vi "TL_Driver_v2.vi"(0 "Device In":refnum<visa-resource-name>="GPIB0::10::INSTR", 5 "Commands":T1(ring)=enum."SET", 7 "Settings":T3={"Module"=enum."WV Online TEC", "WV Online TEC"=23.204500000000476, "WV Online LD"=0.175, "WV Offline TEC"=29.65925000000015, "WV Offline LD"=0.17, "WV Etalon TEC"=30.6, "HSRL Etalon TEC"=25.954, "HSRL TEC"=14.280749999999731, "HSRL LD"=0.16} {"HSRL LD" min=0.0 max=0.18 step=0.001 format="%.3p"; "HSRL TEC" min=14.0 max=28.0 step=0.1 format="%.3g"; "WV Offline LD" min=0.0 max=0.18 step=0.001 format="%.3p"; "WV Online LD" min=0.0 max=0.18 step=0.001 format="%.3p"; "HSRL Etalon TEC" format="%.2g"; "WV Etalon TEC" format="%.2g"; "WV Offline TEC" min=14.0 max=30.0 step=0.1 format="%.3g"; "WV Online TEC" min=14.0 max=28.0 step=0.1 format="%.3g"}, 11 "error in":errorcluster) -> (4 "Device Out":refnum<visa-resource-name>="GPIB0::10::INSTR", 6 "Response":string, 8 "Readings":T2={"Pro8000"=TRUE, "WV OnLine TEC"=23.2082767, "WV Online TEC"=TRUE, "WV Online LD"=0.175123051, "WV Online LD"=TRUE, "WV Offline TEC"=29.6726017, "WV Offline TEC"=TRUE, "WV Offline LD"=0.170392588, "WV Offline LD"=TRUE, "WV EtalonTEC"=30.5354195, "WV Etalon TEC"=TRUE, "HSRL Etalon TEC"=25.9403496, "HSRL Etalon TEC"=TRUE, "HSRL TEC"=14.2948246, "HSRL TEC "=TRUE, "HSRL LD"=0.160259768, "HSRL LD"=TRUE} {"HSRL LD" format="%.3p"; "HSRL TEC" format="%.3g"; "WV Offline LD" format="%.3p"; "WV Online LD" format="%.3p"; "HSRL Etalon TEC" format="%.3g"; "WV EtalonTEC" format="%.3g"; "WV Offline TEC" format="%.3g"; "WV OnLine TEC" format="%.3g"}, 15 "error out":errorcluster)   [LabVIEW 2012]
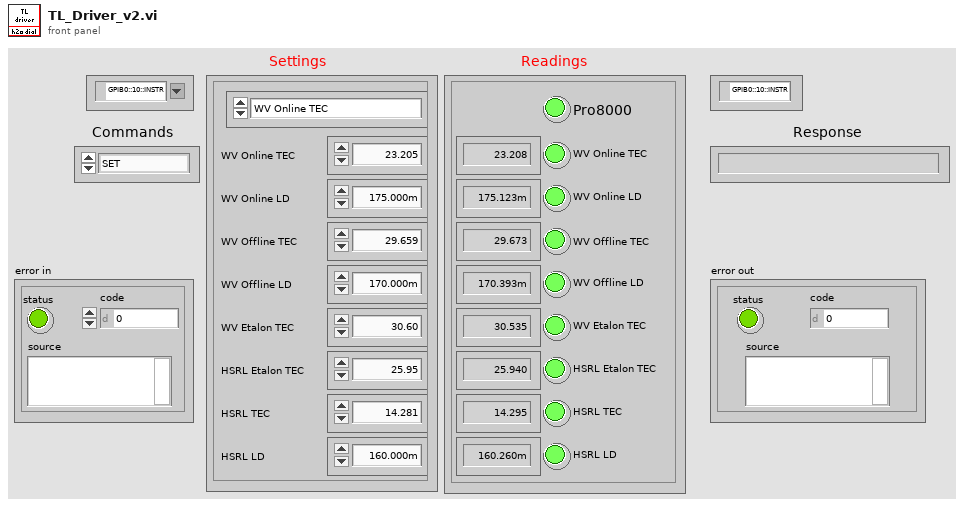
[diagram p1: front panel]
types:
  T1 = enum16{"Open_TL", "Close_TL", "Verify_ID", "TEC_Sensor", "SET", "READ", "ON", "OFF", "Set_Limits", "Read_Limits", "Enable_Status", "Read_Status"}
  T2 = cluster{"Pro8000":bool, "WV OnLine TEC":dbl, "WV Online TEC":bool, "WV Online LD":dbl, "WV Online LD":bool, "WV Offline TEC":dbl, "WV Offline TEC":bool, "WV Offline LD":dbl, "WV Offline LD":bool, "WV EtalonTEC":dbl, "WV Etalon TEC":bool, "HSRL Etalon TEC":dbl, "HSRL Etalon TEC":bool, "HSRL TEC":dbl, "HSRL TEC ":bool, "HSRL LD":dbl, "HSRL LD":bool}
  T3 = cluster{"Module":enum16{"WV Online TEC", "WV Online LD", "WV Offline TEC", "WV Offline LD", "WV Etalon TEC", "HSRL Etalon TEC", "HSRL TEC", "HSRL LD"}, "WV Online TEC":dbl, "WV Online LD":dbl, "WV Offline TEC":dbl, "WV Offline LD":dbl, "WV Etalon TEC":dbl, "HSRL Etalon TEC":dbl, "HSRL TEC":dbl, "HSRL LD":dbl}
  T4 = enum16{"WV Online TEC", "WV Online LD", "WV Offline TEC", "WV Offline LD", "WV Etalon TEC", "HSRL Etalon TEC", "HSRL TEC", "HSRL LD"}
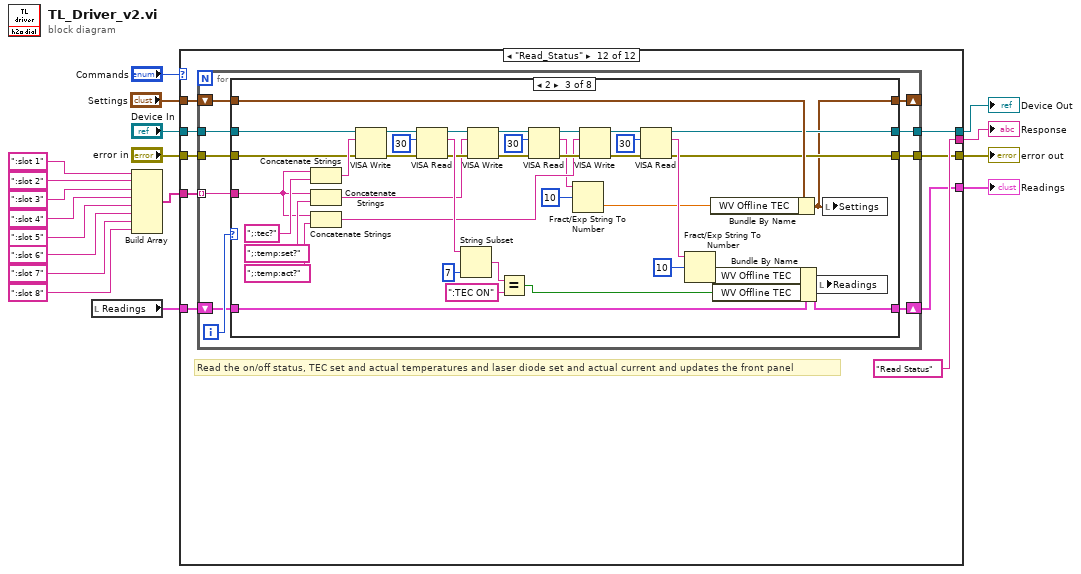
[diagram p0: block diagram]
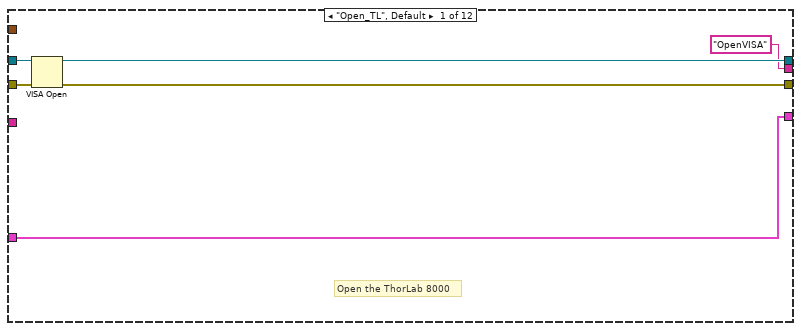
[diagram p2: hidden frame]
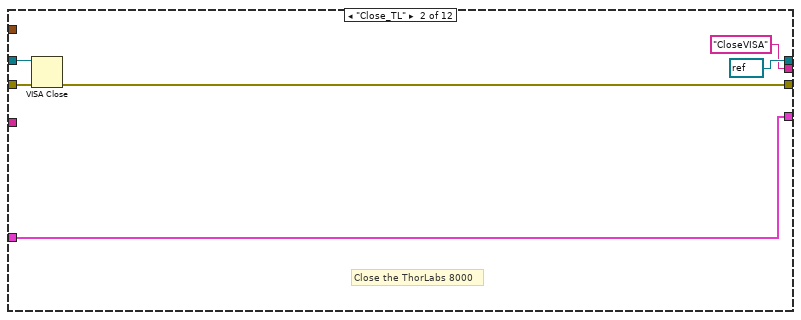
[diagram p3: hidden frame]
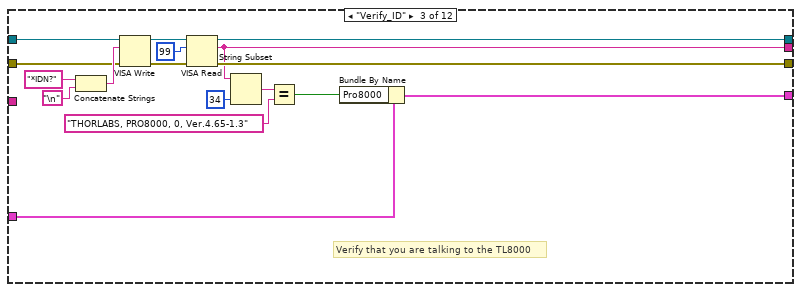
[diagram p4: hidden frame]
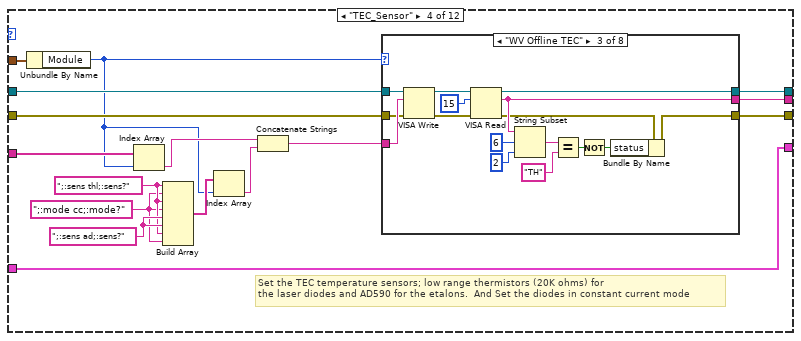
[diagram p5: hidden frame]
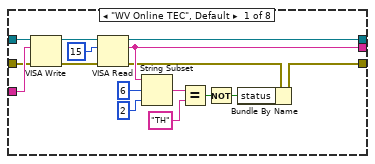
[diagram p6: hidden frame]
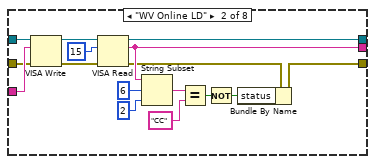
[diagram p7: hidden frame]
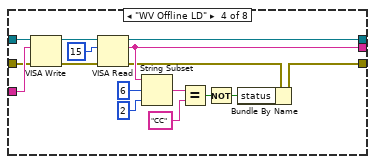
[diagram p8: hidden frame]
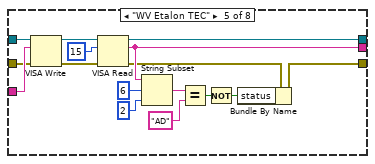
[diagram p9: hidden frame]
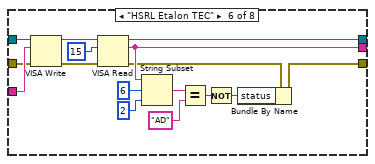
[diagram p10: hidden frame]
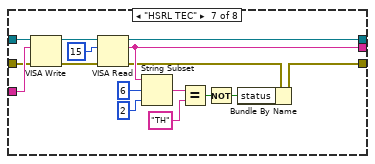
[diagram p11: hidden frame]
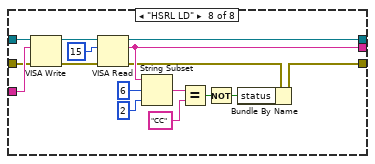
[diagram p12: hidden frame]
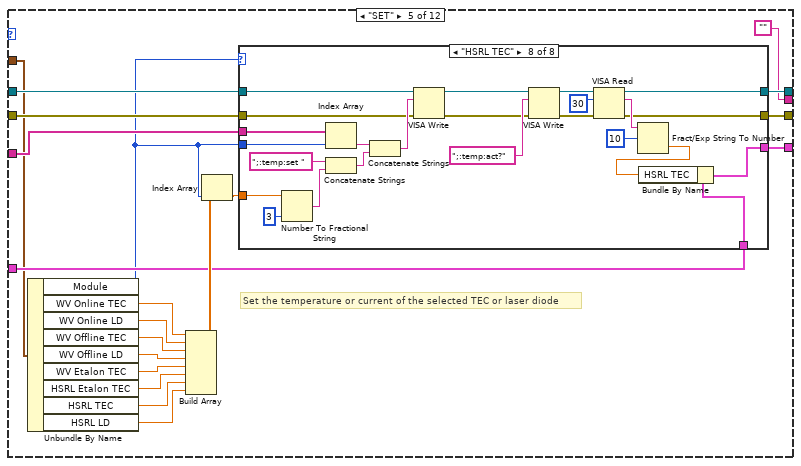
[diagram p13: hidden frame]
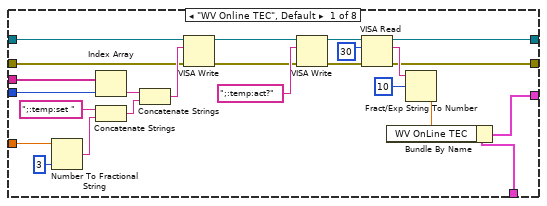
[diagram p14: hidden frame]
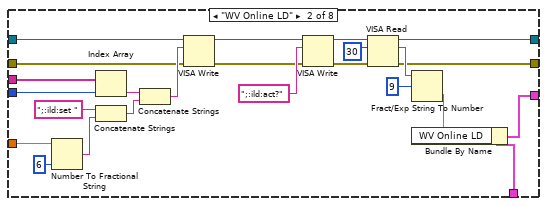
[diagram p15: hidden frame]
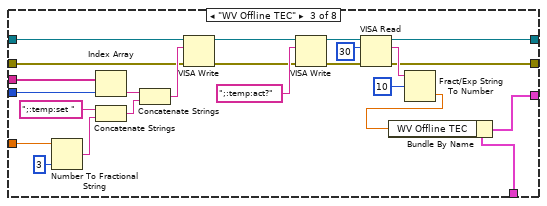
[diagram p16: hidden frame]
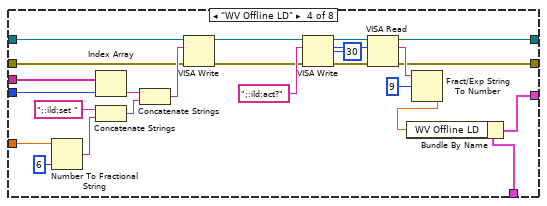
[diagram p17: hidden frame]
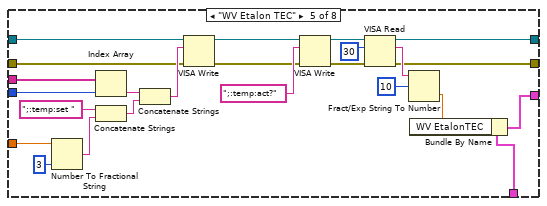
[diagram p18: hidden frame]
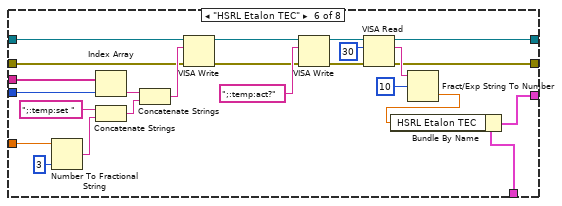
[diagram p19: hidden frame]
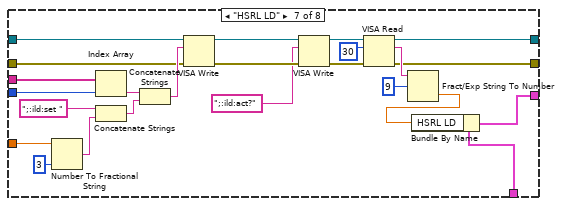
[diagram p20: hidden frame]
diagram:
  n1 = local read "Readings"() -> (w4:T2)
  n2 = Build Array(":slot 1", ":slot 2", ":slot 3", ":slot 4", ":slot 5", ":slot 6", ":slot 7", ":slot 8") -> (w15:string[])
  n3 = case shown="\"Read_Status\"" "Commands" {
    tunnel: "Device In" -> [w24 w30 w44 w62 w211 w418 w538 w698 w852 w856 w860 w867]
    tunnel: "error in" -> [w23 w29 w41 w61 w210 w417 w537 w697 w853 w857 w861 w870]
    tunnel: [w22 refnum<visa-resource-name> refnum ("VISA resource name") w39 w60 w207 w413 w534 w694 w852 w856 w860 w868] -> w13
    tunnel: [w21 w28 w38 w57 w208 w412 w533 w693 w853 w857 w861 w866] -> w17
    tunnel: ["OpenVISA" "CloseVISA" w37 w59 "" "" w532 w692 "" "" "" "Read Status"] -> w12
    tunnel: w15 -> [_ _ _ w56 w209 w415 w535 w695 _ _ _ w871]
    tunnel: "Settings" -> [_ _ _ w55 w201 w411 w531 w691 _ _ _ w869]
    tunnel: w4 -> [w19 w25 w33 w51 w203 w410 w530 w690 w854 w858 w862 w865]
    tunnel: [w19 w25 w32 w51 w202 w409 w529 w689 w854 w858 w862 w864] -> w3
    frame "Open_TL", Default {
      # "Open the ThorLab 8000"
      n4 = VISA Open(error in (no error)=w23, VISA resource name=w24) -> (VISA resource name=w22:refnum<visa-resource-name>, error out=w21:errorcluster)  [unwired: 3 in]
    }
    frame "Close_TL" {
      # "Close the ThorLabs 8000"
      n5 = VISA Close(VISA resource name=w30, error in (no error)=w29) -> (error out=w28:errorcluster)
    }
    frame "Verify_ID" {
      # "Verify that you are talking to the TL8000"
      n6 = Concatenate Strings("*IDN?" ("string"), "\n") -> (w45:string)
      n7 = VISA Write(VISA resource name=w44, write buffer=w45, error in (no error)=w41) -> (VISA resource name out=w42:refnum<visa-resource-name>, error out=w40:errorcluster)  [unwired: 1 out]
      n8 = VISA Read(VISA resource name=w42, byte count=u32 99, error in (no error)=w40) -> (VISA resource name out=w39:refnum<visa-resource-name>, read buffer=w37:string, error out=w38:errorcluster)  [unwired: 1 out]
      n9 = String Subset(string=w37, length (rest)=34 ("length (rest)")) -> (substring=w35:string)  [unwired: 1 in]
      n10 = Equal?(x=w35, y="THORLABS, PRO8000, 0, Ver.4.65-1.3" ("Response")) -> (x = y?=w31:bool)
      n11 = Bundle By Name(cluster=w33, "Pro8000"=w31) -> (w32:T2)
    }
    frame "TEC_Sensor" {
      w48 = ";:mode cc;:mode?"
      w50 = ";:sens ad;:sens?" ("string")
      w49 = ";:sens thl;:sens?" ("string")
      # "Set the TEC temperature sensors; low range thermistors (20K ohms) for\nthe laser diodes and AD590 for the etalons.  And Set the diodes in constant current mode"
      n12 = Unbundle By Name(w55) -> ("Module"=w52:T4)
      n13 = Index Array(array=w56, index=w52) -> (element=w58:string)
      n14 = Build Array(w49, w48, w49, w48, w50, w50, w49, w48) -> (w53:string[])
      n15 = Index Array(array=w53, index=w52) -> (element=w54:string)
      n16 = Concatenate Strings(w58, w54) -> (w63:string)
      n17 = case shown="\"WV Offline TEC\"" w52 {
        tunnel: w63 -> [w79 w95 w111 w127 w143 w159 w175 w191]
        tunnel: w62 -> [w78 w94 w110 w126 w142 w158 w174 w190]
        tunnel: w61 -> [w77 w93 w109 w125 w141 w157 w173 w189]
        tunnel: [w76 w92 w108 w124 w140 w156 w172 w188] -> w60
        tunnel: [w75 w91 w107 w123 w139 w155 w171 w187] -> w59
        tunnel: [w74 w90 w106 w122 w138 w154 w170 w186] -> w57
        frame "WV Online TEC", Default {
          n18 = VISA Write(VISA resource name=w78, write buffer=w79, error in (no error)=w77) -> (VISA resource name out=w66:refnum<visa-resource-name>, error out=w65:errorcluster)  [unwired: 1 out]
          n19 = VISA Read(VISA resource name=w66, byte count=u32 15, error in (no error)=w65) -> (VISA resource name out=w76:refnum<visa-resource-name>, read buffer=w75:string, error out=w72:errorcluster)  [unwired: 1 out]
          n20 = String Subset(string=w75, offset (0)=6 ("length (rest)"), length (rest)=2 ("length (rest)")) -> (substring=w69:string)
          n21 = Equal?(x=w69, y="TH") -> (x = y?=w68:bool)
          n22 = Not(x=w68) -> (.not. x?=w67:bool)
          n23 = Bundle By Name(cluster=w72, "status"=w67) -> (w74:errorcluster)
        }
        frame "WV Online LD" {
          n24 = VISA Write(VISA resource name=w94, write buffer=w95, error in (no error)=w93) -> (VISA resource name out=w82:refnum<visa-resource-name>, error out=w81:errorcluster)  [unwired: 1 out]
          n25 = VISA Read(VISA resource name=w82, byte count=u32 15, error in (no error)=w81) -> (VISA resource name out=w92:refnum<visa-resource-name>, read buffer=w91:string, error out=w88:errorcluster)  [unwired: 1 out]
          n26 = String Subset(string=w91, offset (0)=6 ("length (rest)"), length (rest)=2 ("length (rest)")) -> (substring=w85:string)
          n27 = Equal?(x=w85, y="CC") -> (x = y?=w84:bool)
          n28 = Not(x=w84) -> (.not. x?=w83:bool)
          n29 = Bundle By Name(cluster=w88, "status"=w83) -> (w90:errorcluster)
        }
        frame "WV Offline TEC" {
          n30 = VISA Write(VISA resource name=w110, write buffer=w111, error in (no error)=w109) -> (VISA resource name out=w98:refnum<visa-resource-name>, error out=w97:errorcluster)  [unwired: 1 out]
          n31 = VISA Read(VISA resource name=w98, byte count=u32 15, error in (no error)=w97) -> (VISA resource name out=w108:refnum<visa-resource-name>, read buffer=w107:string, error out=w104:errorcluster)  [unwired: 1 out]
          n32 = String Subset(string=w107, offset (0)=6 ("length (rest)"), length (rest)=2 ("length (rest)")) -> (substring=w101:string)
          n33 = Equal?(x=w101, y="TH") -> (x = y?=w100:bool)
          n34 = Not(x=w100) -> (.not. x?=w99:bool)
          n35 = Bundle By Name(cluster=w104, "status"=w99) -> (w106:errorcluster)
        }
        frame "WV Offline LD" {
          n36 = VISA Write(VISA resource name=w126, write buffer=w127, error in (no error)=w125) -> (VISA resource name out=w114:refnum<visa-resource-name>, error out=w113:errorcluster)  [unwired: 1 out]
          n37 = VISA Read(VISA resource name=w114, byte count=u32 15, error in (no error)=w113) -> (VISA resource name out=w124:refnum<visa-resource-name>, read buffer=w123:string, error out=w120:errorcluster)  [unwired: 1 out]
          n38 = String Subset(string=w123, offset (0)=6 ("length (rest)"), length (rest)=2 ("length (rest)")) -> (substring=w117:string)
          n39 = Equal?(x=w117, y="CC") -> (x = y?=w116:bool)
          n40 = Not(x=w116) -> (.not. x?=w115:bool)
          n41 = Bundle By Name(cluster=w120, "status"=w115) -> (w122:errorcluster)
        }
        frame "WV Etalon TEC" {
          n42 = VISA Write(VISA resource name=w142, write buffer=w143, error in (no error)=w141) -> (VISA resource name out=w130:refnum<visa-resource-name>, error out=w129:errorcluster)  [unwired: 1 out]
          n43 = VISA Read(VISA resource name=w130, byte count=u32 15, error in (no error)=w129) -> (VISA resource name out=w140:refnum<visa-resource-name>, read buffer=w139:string, error out=w136:errorcluster)  [unwired: 1 out]
          n44 = String Subset(string=w139, offset (0)=6 ("length (rest)"), length (rest)=2 ("length (rest)")) -> (substring=w133:string)
          n45 = Equal?(x=w133, y="AD") -> (x = y?=w132:bool)
          n46 = Not(x=w132) -> (.not. x?=w131:bool)
          n47 = Bundle By Name(cluster=w136, "status"=w131) -> (w138:errorcluster)
        }
        frame "HSRL Etalon TEC" {
          n48 = VISA Write(VISA resource name=w158, write buffer=w159, error in (no error)=w157) -> (VISA resource name out=w146:refnum<visa-resource-name>, error out=w145:errorcluster)  [unwired: 1 out]
          n49 = VISA Read(VISA resource name=w146, byte count=u32 15, error in (no error)=w145) -> (VISA resource name out=w156:refnum<visa-resource-name>, read buffer=w155:string, error out=w152:errorcluster)  [unwired: 1 out]
          n50 = String Subset(string=w155, offset (0)=6 ("length (rest)"), length (rest)=2 ("length (rest)")) -> (substring=w149:string)
          n51 = Equal?(x=w149, y="AD") -> (x = y?=w148:bool)
          n52 = Not(x=w148) -> (.not. x?=w147:bool)
          n53 = Bundle By Name(cluster=w152, "status"=w147) -> (w154:errorcluster)
        }
        frame "HSRL TEC" {
          n54 = VISA Write(VISA resource name=w174, write buffer=w175, error in (no error)=w173) -> (VISA resource name out=w162:refnum<visa-resource-name>, error out=w161:errorcluster)  [unwired: 1 out]
          n55 = VISA Read(VISA resource name=w162, byte count=u32 15, error in (no error)=w161) -> (VISA resource name out=w172:refnum<visa-resource-name>, read buffer=w171:string, error out=w168:errorcluster)  [unwired: 1 out]
          n56 = String Subset(string=w171, offset (0)=6 ("length (rest)"), length (rest)=2 ("length (rest)")) -> (substring=w165:string)
          n57 = Equal?(x=w165, y="TH") -> (x = y?=w164:bool)
          n58 = Not(x=w164) -> (.not. x?=w163:bool)
          n59 = Bundle By Name(cluster=w168, "status"=w163) -> (w170:errorcluster)
        }
        frame "HSRL LD" {
          n60 = VISA Write(VISA resource name=w190, write buffer=w191, error in (no error)=w189) -> (VISA resource name out=w178:refnum<visa-resource-name>, error out=w177:errorcluster)  [unwired: 1 out]
          n61 = VISA Read(VISA resource name=w178, byte count=u32 15, error in (no error)=w177) -> (VISA resource name out=w188:refnum<visa-resource-name>, read buffer=w187:string, error out=w184:errorcluster)  [unwired: 1 out]
          n62 = String Subset(string=w187, offset (0)=6 ("length (rest)"), length (rest)=2 ("length (rest)")) -> (substring=w181:string)
          n63 = Equal?(x=w181, y="CC") -> (x = y?=w180:bool)
          n64 = Not(x=w180) -> (.not. x?=w179:bool)
          n65 = Bundle By Name(cluster=w184, "status"=w179) -> (w186:errorcluster)
        }
      }
    }
    frame "SET" {
      # "Set the temperature or current of the selected TEC or laser diode"
      n66 = Unbundle By Name(w201) -> ("Module"=w192:T4, "WV Online TEC"=w200:dbl, "WV Online LD"=w199:dbl, "WV Offline TEC"=w198:dbl, "WV Offline LD"=w193:dbl, "WV Etalon TEC"=w194:dbl, "HSRL Etalon TEC"=w197:dbl, "HSRL TEC"=w196:dbl, "HSRL LD"=w195:dbl)
      n67 = Build Array(w200, w199, w198, w193, w194, w197, w196, w195) -> (w205:dbl[])
      n68 = Index Array(array=w205, index=w192) -> (element=w204:dbl)
      n69 = case shown="\"HSRL TEC\"" w192 {
        tunnel: w211 -> [w234 w258 w282 w306 w330 w354 w378 w402]
        tunnel: w210 -> [w233 w257 w281 w305 w329 w353 w377 w401]
        tunnel: w209 -> [w231 w255 w279 w303 w327 w351 w375 w399]
        tunnel: [w216 w242 w265 w289 w312 w336 w362 w384] -> w208
        tunnel: [w215 w241 w263 w288 w311 w335 w361 w383] -> w207
        tunnel: w204 -> [w225 w249 w273 w297 w321 w345 w370 w393]
        tunnel: w192 -> [w226 w250 w274 w298 w322 w346 w371 w394]
        tunnel: w203 -> [w218 w239 w267 w287 w313 w338 w364 w386]
        tunnel: [w217 w238 w266 w286 w314 w339 w365 w387] -> w202
        frame "WV Online TEC", Default {
          n70 = Number To Fractional String(number=w225, precision (6)=i16 3) -> (F-format string=w230:string)  [unwired: 2 in]
          n71 = Index Array(array=w231, index=w226) -> (element=w232:string)
          n72 = Concatenate Strings(";:temp:set " ("write buffer"), w230) -> (w227:string)
          n73 = Concatenate Strings(w232, w227) -> (w235:string)
          n74 = VISA Write(VISA resource name=w234, write buffer=w235, error in (no error)=w233) -> (VISA resource name out=w213:refnum<visa-resource-name>, error out=w212:errorcluster)  [unwired: 1 out]
          n75 = VISA Write(VISA resource name=w213, write buffer=";:temp:act?", error in (no error)=w212) -> (VISA resource name out=w220:refnum<visa-resource-name>, error out=w221:errorcluster)  [unwired: 1 out]
          n76 = VISA Read(VISA resource name=w220, byte count=u32 30, error in (no error)=w221) -> (VISA resource name out=w215:refnum<visa-resource-name>, read buffer=w222:string, error out=w216:errorcluster)  [unwired: 1 out]
          n77 = Fract/Exp String To Number(string=w222, offset=10) -> (number=w219:dbl)  [unwired: 2 in, 1 out]
          n78 = Bundle By Name(cluster=w218, "WV OnLine TEC"=w219) -> (w217:T2)
        }
        frame "WV Online LD" {
          n79 = Number To Fractional String(number=w249, precision (6)=i16 6) -> (F-format string=w254:string)  [unwired: 2 in]
          n80 = Index Array(array=w255, index=w250) -> (element=w256:string)
          n81 = Concatenate Strings(";:ild:set " ("write buffer"), w254) -> (w251:string)
          n82 = Concatenate Strings(w256, w251) -> (w259:string)
          n83 = VISA Write(VISA resource name=w258, write buffer=w259, error in (no error)=w257) -> (VISA resource name out=w237:refnum<visa-resource-name>, error out=w236:errorcluster)  [unwired: 1 out]
          n84 = VISA Write(VISA resource name=w237, write buffer=";:ild:act?", error in (no error)=w236) -> (VISA resource name out=w244:refnum<visa-resource-name>, error out=w245:errorcluster)  [unwired: 1 out]
          n85 = VISA Read(VISA resource name=w244, byte count=u32 30, error in (no error)=w245) -> (VISA resource name out=w241:refnum<visa-resource-name>, read buffer=w246:string, error out=w242:errorcluster)  [unwired: 1 out]
          n86 = Fract/Exp String To Number(string=w246, offset=9) -> (number=w243:dbl)  [unwired: 2 in, 1 out]
          n87 = Bundle By Name(cluster=w239, "WV Online LD"=w243) -> (w238:T2)
        }
        frame "WV Offline TEC" {
          n88 = Number To Fractional String(number=w273, precision (6)=i16 3) -> (F-format string=w278:string)  [unwired: 2 in]
          n89 = Index Array(array=w279, index=w274) -> (element=w280:string)
          n90 = Concatenate Strings(";:temp:set " ("write buffer"), w278) -> (w275:string)
          n91 = Concatenate Strings(w280, w275) -> (w283:string)
          n92 = VISA Write(VISA resource name=w282, write buffer=w283, error in (no error)=w281) -> (VISA resource name out=w262:refnum<visa-resource-name>, error out=w261:errorcluster)  [unwired: 1 out]
          n93 = VISA Write(VISA resource name=w262, write buffer=";:temp:act?", error in (no error)=w261) -> (VISA resource name out=w264:refnum<visa-resource-name>, error out=w269:errorcluster)  [unwired: 1 out]
          n94 = VISA Read(VISA resource name=w264, byte count=u32 30, error in (no error)=w269) -> (VISA resource name out=w263:refnum<visa-resource-name>, read buffer=w270:string, error out=w265:errorcluster)  [unwired: 1 out]
          n95 = Fract/Exp String To Number(string=w270, offset=10) -> (number=w260:dbl)  [unwired: 2 in, 1 out]
          n96 = Bundle By Name(cluster=w267, "WV Offline TEC"=w260) -> (w266:T2)
        }
        frame "WV Offline LD" {
          n97 = Number To Fractional String(number=w297, precision (6)=i16 6) -> (F-format string=w302:string)  [unwired: 2 in]
          n98 = Index Array(array=w303, index=w298) -> (element=w304:string)
          n99 = Concatenate Strings(";:ild:set " ("write buffer"), w302) -> (w299:string)
          n100 = Concatenate Strings(w304, w299) -> (w307:string)
          n101 = VISA Write(VISA resource name=w306, write buffer=w307, error in (no error)=w305) -> (VISA resource name out=w285:refnum<visa-resource-name>, error out=w284:errorcluster)  [unwired: 1 out]
          n102 = VISA Write(VISA resource name=w285, write buffer=";:ild:act?", error in (no error)=w284) -> (VISA resource name out=w292:refnum<visa-resource-name>, error out=w293:errorcluster)  [unwired: 1 out]
          n103 = VISA Read(VISA resource name=w292, byte count=u32 30, error in (no error)=w293) -> (VISA resource name out=w288:refnum<visa-resource-name>, read buffer=w294:string, error out=w289:errorcluster)  [unwired: 1 out]
          n104 = Fract/Exp String To Number(string=w294, offset=9) -> (number=w291:dbl)  [unwired: 2 in, 1 out]
          n105 = Bundle By Name(cluster=w287, "WV Offline LD"=w291) -> (w286:T2)
        }
        frame "WV Etalon TEC" {
          n106 = Number To Fractional String(number=w321, precision (6)=i16 3) -> (F-format string=w326:string)  [unwired: 2 in]
          n107 = Index Array(array=w327, index=w322) -> (element=w328:string)
          n108 = Concatenate Strings(";:temp:set " ("write buffer"), w326) -> (w323:string)
          n109 = Concatenate Strings(w328, w323) -> (w331:string)
          n110 = VISA Write(VISA resource name=w330, write buffer=w331, error in (no error)=w329) -> (VISA resource name out=w309:refnum<visa-resource-name>, error out=w308:errorcluster)  [unwired: 1 out]
          n111 = VISA Write(VISA resource name=w309, write buffer=";:temp:act?", error in (no error)=w308) -> (VISA resource name out=w310:refnum<visa-resource-name>, error out=w317:errorcluster)  [unwired: 1 out]
          n112 = VISA Read(VISA resource name=w310, byte count=u32 30, error in (no error)=w317) -> (VISA resource name out=w311:refnum<visa-resource-name>, read buffer=w318:string, error out=w312:errorcluster)  [unwired: 1 out]
          n113 = Fract/Exp String To Number(string=w318, offset=10) -> (number=w316:dbl)  [unwired: 2 in, 1 out]
          n114 = Bundle By Name(cluster=w313, "WV EtalonTEC"=w316) -> (w314:T2)
        }
        frame "HSRL Etalon TEC" {
          n115 = Number To Fractional String(number=w345, precision (6)=i16 3) -> (F-format string=w350:string)  [unwired: 2 in]
          n116 = Index Array(array=w351, index=w346) -> (element=w352:string)
          n117 = Concatenate Strings(";:temp:set " ("write buffer"), w350) -> (w347:string)
          n118 = Concatenate Strings(w352, w347) -> (w355:string)
          n119 = VISA Write(VISA resource name=w354, write buffer=w355, error in (no error)=w353) -> (VISA resource name out=w334:refnum<visa-resource-name>, error out=w333:errorcluster)  [unwired: 1 out]
          n120 = VISA Write(VISA resource name=w334, write buffer=";:temp:act?", error in (no error)=w333) -> (VISA resource name out=w337:refnum<visa-resource-name>, error out=w341:errorcluster)  [unwired: 1 out]
          n121 = VISA Read(VISA resource name=w337, byte count=u32 30, error in (no error)=w341) -> (VISA resource name out=w335:refnum<visa-resource-name>, read buffer=w342:string, error out=w336:errorcluster)  [unwired: 1 out]
          n122 = Fract/Exp String To Number(string=w342, offset=10) -> (number=w332:dbl)  [unwired: 2 in, 1 out]
          n123 = Bundle By Name(cluster=w338, "HSRL Etalon TEC"=w332) -> (w339:T2)
        }
        frame "HSRL LD" {
          n124 = Number To Fractional String(number=w370, precision (6)=i16 3) -> (F-format string=w374:string)  [unwired: 2 in]
          n125 = Index Array(array=w375, index=w371) -> (element=w376:string)
          n126 = Concatenate Strings(";:ild:set " ("write buffer"), w374) -> (w372:string)
          n127 = Concatenate Strings(w376, w372) -> (w379:string)
          n128 = VISA Write(VISA resource name=w378, write buffer=w379, error in (no error)=w377) -> (VISA resource name out=w360:refnum<visa-resource-name>, error out=w359:errorcluster)  [unwired: 1 out]
          n129 = VISA Write(VISA resource name=w360, write buffer=";:ild:act?", error in (no error)=w359) -> (VISA resource name out=w363:refnum<visa-resource-name>, error out=w366:errorcluster)  [unwired: 1 out]
          n130 = VISA Read(VISA resource name=w363, byte count=u32 30, error in (no error)=w366) -> (VISA resource name out=w361:refnum<visa-resource-name>, read buffer=w367:string, error out=w362:errorcluster)  [unwired: 1 out]
          n131 = Fract/Exp String To Number(string=w367, offset=9) -> (number=w358:dbl)  [unwired: 2 in, 1 out]
          n132 = Bundle By Name(cluster=w364, "HSRL LD"=w358) -> (w365:T2)
        }
        frame "HSRL TEC" {
          n133 = Number To Fractional String(number=w393, precision (6)=i16 3) -> (F-format string=w398:string)  [unwired: 2 in]
          n134 = Index Array(array=w399, index=w394) -> (element=w400:string)
          n135 = Concatenate Strings(";:temp:set " ("write buffer"), w398) -> (w395:string)
          n136 = Concatenate Strings(w400, w395) -> (w403:string)
          n137 = VISA Write(VISA resource name=w402, write buffer=w403, error in (no error)=w401) -> (VISA resource name out=w382:refnum<visa-resource-name>, error out=w381:errorcluster)  [unwired: 1 out]
          n138 = VISA Write(VISA resource name=w382, write buffer=";:temp:act?", error in (no error)=w381) -> (VISA resource name out=w385:refnum<visa-resource-name>, error out=w389:errorcluster)  [unwired: 1 out]
          n139 = VISA Read(VISA resource name=w385, byte count=u32 30, error in (no error)=w389) -> (VISA resource name out=w383:refnum<visa-resource-name>, read buffer=w390:string, error out=w384:errorcluster)  [unwired: 1 out]
          n140 = Fract/Exp String To Number(string=w390, offset=10) -> (number=w380:dbl)  [unwired: 2 in, 1 out]
          n141 = Bundle By Name(cluster=w386, "HSRL TEC"=w380) -> (w387:T2)
        }
      }
    }
    frame "READ" {
      w406 = ";:ild:act? " ("write buffer")
      w405 = ";:temp:act? " ("write buffer")
      # "Read the actual temp or current of the selected TEC or laser diodes"
      n142 = Unbundle By Name(w411) -> ("Module"=w408:T4)
      n143 = Index Array(array=w415, index=w408) -> (element=w416:string)
      n144 = Build Array(w405, w406, w405, w406, w405, w405, w405, w406) -> (w404:string[])
      n145 = Index Array(array=w404, index=w408) -> (element=w407:string)
      n146 = Concatenate Strings(w416, w407) -> (w419:string)
      n147 = case shown="\"HSRL TEC\"" w408 {
        tunnel: w419 -> [w432 w445 w458 w471 w484 w497 w510 w523]
        tunnel: w418 -> [w431 w444 w457 w470 w483 w496 w509 w522]
        tunnel: w417 -> [w430 w443 w456 w469 w482 w495 w508 w521]
        tunnel: [w424 w437 w450 w463 w476 w489 w502 w515] -> w413
        tunnel: [w423 w436 w449 w462 w475 w488 w501 w514] -> w412
        tunnel: w410 -> [w421 w434 w447 w460 w473 w486 w499 w512]
        tunnel: [w420 w433 w446 w459 w472 w485 w498 w511] -> w409
        frame "WV Online TEC", Default {
          n148 = VISA Write(VISA resource name=w431, write buffer=w432, error in (no error)=w430) -> (VISA resource name out=w425:refnum<visa-resource-name>, error out=w426:errorcluster)  [unwired: 1 out]
          n149 = VISA Read(VISA resource name=w425, byte count=u32 30, error in (no error)=w426) -> (VISA resource name out=w424:refnum<visa-resource-name>, read buffer=w427:string, error out=w423:errorcluster)  [unwired: 1 out]
          n150 = Fract/Exp String To Number(string=w427, offset=10) -> (number=w422:dbl)  [unwired: 2 in, 1 out]
          n151 = Bundle By Name(cluster=w421, "WV OnLine TEC"=w422) -> (w420:T2)
        }
        frame "WV Online LD" {
          n152 = VISA Write(VISA resource name=w444, write buffer=w445, error in (no error)=w443) -> (VISA resource name out=w438:refnum<visa-resource-name>, error out=w439:errorcluster)  [unwired: 1 out]
          n153 = VISA Read(VISA resource name=w438, byte count=u32 30, error in (no error)=w439) -> (VISA resource name out=w437:refnum<visa-resource-name>, read buffer=w440:string, error out=w436:errorcluster)  [unwired: 1 out]
          n154 = Fract/Exp String To Number(string=w440, offset=9) -> (number=w435:dbl)  [unwired: 2 in, 1 out]
          n155 = Bundle By Name(cluster=w434, "WV Online LD"=w435) -> (w433:T2)
        }
        frame "WV Offline TEC" {
          n156 = VISA Write(VISA resource name=w457, write buffer=w458, error in (no error)=w456) -> (VISA resource name out=w451:refnum<visa-resource-name>, error out=w452:errorcluster)  [unwired: 1 out]
          n157 = VISA Read(VISA resource name=w451, byte count=u32 30, error in (no error)=w452) -> (VISA resource name out=w450:refnum<visa-resource-name>, read buffer=w453:string, error out=w449:errorcluster)  [unwired: 1 out]
          n158 = Fract/Exp String To Number(string=w453, offset=10) -> (number=w448:dbl)  [unwired: 2 in, 1 out]
          n159 = Bundle By Name(cluster=w447, "WV Offline TEC"=w448) -> (w446:T2)
        }
        frame "WV Offline LD" {
          n160 = VISA Write(VISA resource name=w470, write buffer=w471, error in (no error)=w469) -> (VISA resource name out=w464:refnum<visa-resource-name>, error out=w465:errorcluster)  [unwired: 1 out]
          n161 = VISA Read(VISA resource name=w464, byte count=u32 30, error in (no error)=w465) -> (VISA resource name out=w463:refnum<visa-resource-name>, read buffer=w466:string, error out=w462:errorcluster)  [unwired: 1 out]
          n162 = Fract/Exp String To Number(string=w466, offset=9) -> (number=w461:dbl)  [unwired: 2 in, 1 out]
          n163 = Bundle By Name(cluster=w460, "WV Offline LD"=w461) -> (w459:T2)
        }
        frame "WV Etalon TEC" {
          n164 = VISA Write(VISA resource name=w483, write buffer=w484, error in (no error)=w482) -> (VISA resource name out=w477:refnum<visa-resource-name>, error out=w478:errorcluster)  [unwired: 1 out]
          n165 = VISA Read(VISA resource name=w477, byte count=u32 30, error in (no error)=w478) -> (VISA resource name out=w476:refnum<visa-resource-name>, read buffer=w479:string, error out=w475:errorcluster)  [unwired: 1 out]
          n166 = Fract/Exp String To Number(string=w479, offset=10) -> (number=w474:dbl)  [unwired: 2 in, 1 out]
          n167 = Bundle By Name(cluster=w473, "WV EtalonTEC"=w474) -> (w472:T2)
        }
        frame "HSRL Etalon TEC" {
          n168 = VISA Write(VISA resource name=w496, write buffer=w497, error in (no error)=w495) -> (VISA resource name out=w490:refnum<visa-resource-name>, error out=w491:errorcluster)  [unwired: 1 out]
          n169 = VISA Read(VISA resource name=w490, byte count=u32 30, error in (no error)=w491) -> (VISA resource name out=w489:refnum<visa-resource-name>, read buffer=w492:string, error out=w488:errorcluster)  [unwired: 1 out]
          n170 = Fract/Exp String To Number(string=w492, offset=10) -> (number=w487:dbl)  [unwired: 2 in, 1 out]
          n171 = Bundle By Name(cluster=w486, "HSRL Etalon TEC"=w487) -> (w485:T2)
        }
        frame "HSRL TEC" {
          n172 = VISA Write(VISA resource name=w509, write buffer=w510, error in (no error)=w508) -> (VISA resource name out=w503:refnum<visa-resource-name>, error out=w504:errorcluster)  [unwired: 1 out]
          n173 = VISA Read(VISA resource name=w503, byte count=u32 30, error in (no error)=w504) -> (VISA resource name out=w502:refnum<visa-resource-name>, read buffer=w505:string, error out=w501:errorcluster)  [unwired: 1 out]
          n174 = Fract/Exp String To Number(string=w505, offset=10) -> (number=w500:dbl)  [unwired: 2 in, 1 out]
          n175 = Bundle By Name(cluster=w499, "HSRL TEC"=w500) -> (w498:T2)
        }
        frame "HSRL LD" {
          n176 = VISA Write(VISA resource name=w522, write buffer=w523, error in (no error)=w521) -> (VISA resource name out=w516:refnum<visa-resource-name>, error out=w517:errorcluster)  [unwired: 1 out]
          n177 = VISA Read(VISA resource name=w516, byte count=u32 30, error in (no error)=w517) -> (VISA resource name out=w515:refnum<visa-resource-name>, read buffer=w518:string, error out=w514:errorcluster)  [unwired: 1 out]
          n178 = Fract/Exp String To Number(string=w518, offset=9) -> (number=w513:dbl)  [unwired: 2 in, 1 out]
          n179 = Bundle By Name(cluster=w512, "HSRL LD"=w513) -> (w511:T2)
        }
      }
    }
    frame "ON" {
      w525 = ";:laser on" ("write buffer")
      w524 = ";:tec on" ("write buffer")
      # "Turn the selected TEC or laser on"
      n180 = Unbundle By Name(w531) -> ("Module"=w527:T4)
      n181 = Build Array(w524, w525, w524, w525, w524, w524, w524, w525) -> (w528:string[])
      n182 = Index Array(array=w535, index=w527) -> (element=w536:string)
      n183 = Index Array(array=w528, index=w527) -> (element=w526:string)
      n184 = Concatenate Strings(w536, w526) -> (w539:string)
      n185 = case shown="\"HSRL Etalon TEC\"" w527 {
        tunnel: w539 -> [w557 w575 w593 w611 w629 w647 w665 w683]
        tunnel: w538 -> [w556 w574 w592 w610 w628 w646 w664 w682]
        tunnel: w537 -> [w555 w573 w591 w609 w627 w645 w663 w681]
        tunnel: [w553 w571 w589 w607 w625 w643 w661 w679] -> w534
        tunnel: [w552 w570 w588 w606 w624 w642 w660 w678] -> w533
        tunnel: [w543 w561 w579 w597 w615 w633 w651 w671] -> w532
        tunnel: w530 -> [w542 w560 w578 w596 w614 w632 w650 w670]
        tunnel: [w541 w559 w577 w595 w613 w631 w649 w669] -> w529
        frame "WV Online TEC", Default {
          n186 = VISA Write(VISA resource name=w556, write buffer=w557, error in (no error)=w555) -> (VISA resource name out=w549:refnum<visa-resource-name>, error out=w551:errorcluster)  [unwired: 1 out]
          n187 = VISA Write(VISA resource name=w549, write buffer=":tec?", error in (no error)=w551) -> (VISA resource name out=w548:refnum<visa-resource-name>, error out=w550:errorcluster)  [unwired: 1 out]
          n188 = VISA Read(VISA resource name=w548, byte count=u32 15, error in (no error)=w550) -> (VISA resource name out=w553:refnum<visa-resource-name>, read buffer=w543:string, error out=w552:errorcluster)  [unwired: 1 out]
          n189 = String Subset(string=w543, length (rest)=7 ("offset (0)")) -> (substring=w545:string)  [unwired: 1 in]
          n190 = Equal?(x=w545, y=":TEC ON") -> (x = y?=w540:bool)
          n191 = Bundle By Name(cluster=w542, "WV Online TEC"=w540) -> (w541:T2)
        }
        frame "WV Online LD" {
          n192 = VISA Write(VISA resource name=w574, write buffer=w575, error in (no error)=w573) -> (VISA resource name out=w567:refnum<visa-resource-name>, error out=w569:errorcluster)  [unwired: 1 out]
          n193 = VISA Write(VISA resource name=w567, write buffer=":laser?", error in (no error)=w569) -> (VISA resource name out=w566:refnum<visa-resource-name>, error out=w568:errorcluster)  [unwired: 1 out]
          n194 = VISA Read(VISA resource name=w566, byte count=u32 15, error in (no error)=w568) -> (VISA resource name out=w571:refnum<visa-resource-name>, read buffer=w561:string, error out=w570:errorcluster)  [unwired: 1 out]
          n195 = String Subset(string=w561, length (rest)=9 ("offset (0)")) -> (substring=w563:string)  [unwired: 1 in]
          n196 = Equal?(x=w563, y=":LASER ON") -> (x = y?=w558:bool)
          n197 = Bundle By Name(cluster=w560, "WV Online LD"=w558) -> (w559:T2)
        }
        frame "WV Offline TEC" {
          n198 = VISA Write(VISA resource name=w592, write buffer=w593, error in (no error)=w591) -> (VISA resource name out=w585:refnum<visa-resource-name>, error out=w587:errorcluster)  [unwired: 1 out]
          n199 = VISA Write(VISA resource name=w585, write buffer=":tec?", error in (no error)=w587) -> (VISA resource name out=w584:refnum<visa-resource-name>, error out=w586:errorcluster)  [unwired: 1 out]
          n200 = VISA Read(VISA resource name=w584, byte count=u32 15, error in (no error)=w586) -> (VISA resource name out=w589:refnum<visa-resource-name>, read buffer=w579:string, error out=w588:errorcluster)  [unwired: 1 out]
          n201 = String Subset(string=w579, length (rest)=7 ("offset (0)")) -> (substring=w581:string)  [unwired: 1 in]
          n202 = Equal?(x=w581, y=":TEC ON") -> (x = y?=w576:bool)
          n203 = Bundle By Name(cluster=w578, "WV Offline TEC"=w576) -> (w577:T2)
        }
        frame "WV Offline LD" {
          n204 = VISA Write(VISA resource name=w610, write buffer=w611, error in (no error)=w609) -> (VISA resource name out=w603:refnum<visa-resource-name>, error out=w605:errorcluster)  [unwired: 1 out]
          n205 = VISA Write(VISA resource name=w603, write buffer=":laser?", error in (no error)=w605) -> (VISA resource name out=w602:refnum<visa-resource-name>, error out=w604:errorcluster)  [unwired: 1 out]
          n206 = VISA Read(VISA resource name=w602, byte count=u32 15, error in (no error)=w604) -> (VISA resource name out=w607:refnum<visa-resource-name>, read buffer=w597:string, error out=w606:errorcluster)  [unwired: 1 out]
          n207 = String Subset(string=w597, length (rest)=9 ("offset (0)")) -> (substring=w599:string)  [unwired: 1 in]
          n208 = Equal?(x=w599, y=":LASER ON") -> (x = y?=w594:bool)
          n209 = Bundle By Name(cluster=w596, "WV Offline LD"=w594) -> (w595:T2)
        }
        frame "WV Etalon TEC" {
          n210 = VISA Write(VISA resource name=w628, write buffer=w629, error in (no error)=w627) -> (VISA resource name out=w621:refnum<visa-resource-name>, error out=w623:errorcluster)  [unwired: 1 out]
          n211 = VISA Write(VISA resource name=w621, write buffer=":tec?", error in (no error)=w623) -> (VISA resource name out=w620:refnum<visa-resource-name>, error out=w622:errorcluster)  [unwired: 1 out]
          n212 = VISA Read(VISA resource name=w620, byte count=u32 15, error in (no error)=w622) -> (VISA resource name out=w625:refnum<visa-resource-name>, read buffer=w615:string, error out=w624:errorcluster)  [unwired: 1 out]
          n213 = String Subset(string=w615, length (rest)=7 ("offset (0)")) -> (substring=w617:string)  [unwired: 1 in]
          n214 = Equal?(x=w617, y=":TEC ON") -> (x = y?=w612:bool)
          n215 = Bundle By Name(cluster=w614, "WV Etalon TEC"=w612) -> (w613:T2)
        }
        frame "HSRL Etalon TEC" {
          n216 = VISA Write(VISA resource name=w646, write buffer=w647, error in (no error)=w645) -> (VISA resource name out=w639:refnum<visa-resource-name>, error out=w641:errorcluster)  [unwired: 1 out]
          n217 = VISA Write(VISA resource name=w639, write buffer=":tec?", error in (no error)=w641) -> (VISA resource name out=w638:refnum<visa-resource-name>, error out=w640:errorcluster)  [unwired: 1 out]
          n218 = VISA Read(VISA resource name=w638, byte count=u32 15, error in (no error)=w640) -> (VISA resource name out=w643:refnum<visa-resource-name>, read buffer=w633:string, error out=w642:errorcluster)  [unwired: 1 out]
          n219 = String Subset(string=w633, length (rest)=7 ("offset (0)")) -> (substring=w635:string)  [unwired: 1 in]
          n220 = Equal?(x=w635, y=":TEC ON") -> (x = y?=w630:bool)
          n221 = Bundle By Name(cluster=w632, "HSRL Etalon TEC"=w630) -> (w631:T2)
        }
        frame "HSRL TEC" {
          n222 = VISA Write(VISA resource name=w664, write buffer=w665, error in (no error)=w663) -> (VISA resource name out=w657:refnum<visa-resource-name>, error out=w659:errorcluster)  [unwired: 1 out]
          n223 = VISA Write(VISA resource name=w657, write buffer=":tec?", error in (no error)=w659) -> (VISA resource name out=w656:refnum<visa-resource-name>, error out=w658:errorcluster)  [unwired: 1 out]
          n224 = VISA Read(VISA resource name=w656, byte count=u32 15, error in (no error)=w658) -> (VISA resource name out=w661:refnum<visa-resource-name>, read buffer=w651:string, error out=w660:errorcluster)  [unwired: 1 out]
          n225 = String Subset(string=w651, length (rest)=7 ("offset (0)")) -> (substring=w653:string)  [unwired: 1 in]
          n226 = Equal?(x=w653, y=":TEC ON") -> (x = y?=w648:bool)
          n227 = Bundle By Name(cluster=w650, "HSRL TEC"=w648) -> (w649:T2)
        }
        frame "HSRL LD" {
          n228 = VISA Write(VISA resource name=w682, write buffer=w683, error in (no error)=w681) -> (VISA resource name out=w675:refnum<visa-resource-name>, error out=w677:errorcluster)  [unwired: 1 out]
          n229 = VISA Write(VISA resource name=w675, write buffer=":laser?", error in (no error)=w677) -> (VISA resource name out=w674:refnum<visa-resource-name>, error out=w676:errorcluster)  [unwired: 1 out]
          n230 = VISA Read(VISA resource name=w674, byte count=u32 15, error in (no error)=w676) -> (VISA resource name out=w679:refnum<visa-resource-name>, read buffer=w671:string, error out=w678:errorcluster)  [unwired: 1 out]
          n231 = String Subset(string=w671, length (rest)=9 ("offset (0)")) -> (substring=w673:string)  [unwired: 1 in]
          n232 = Equal?(x=w673, y=":LASER ON") -> (x = y?=w668:bool)
          n233 = Bundle By Name(cluster=w670, "HSRL LD"=w668) -> (w669:T2)
        }
      }
    }
    frame "OFF" {
      w684 = ";:laser off" ("write buffer")
      w685 = ";:tec off" ("write buffer")
      # "Turn the selected TEC or laser off"
      n234 = Unbundle By Name(w691) -> ("Module"=w686:T4)
      n235 = Build Array(w685, w684, w685, w684, w685, w685, w685, w684) -> (w688:string[])
      n236 = Index Array(array=w695, index=w686) -> (element=w696:string)
      n237 = Index Array(array=w688, index=w686) -> (element=w687:string)
      n238 = Concatenate Strings(w696, w687) -> (w699:string)
      n239 = case shown="\"HSRL TEC\"" w686 {
        tunnel: w699 -> [w718 w737 w756 w775 w794 w813 w832 w851]
        tunnel: w698 -> [w717 w736 w755 w774 w793 w812 w831 w850]
        tunnel: w697 -> [w716 w735 w754 w773 w792 w811 w830 w849]
        tunnel: [w714 w733 w752 w771 w790 w809 w828 w847] -> w694
        tunnel: [w713 w732 w751 w770 w789 w808 w827 w846] -> w693
        tunnel: [w704 w723 w742 w761 w780 w799 w818 w839] -> w692
        tunnel: w690 -> [w703 w722 w741 w760 w779 w798 w817 w838]
        tunnel: [w702 w721 w740 w759 w778 w797 w816 w837] -> w689
        frame "WV Online TEC", Default {
          n240 = VISA Write(VISA resource name=w717, write buffer=w718, error in (no error)=w716) -> (VISA resource name out=w710:refnum<visa-resource-name>, error out=w712:errorcluster)  [unwired: 1 out]
          n241 = VISA Write(VISA resource name=w710, write buffer=":tec?", error in (no error)=w712) -> (VISA resource name out=w709:refnum<visa-resource-name>, error out=w711:errorcluster)  [unwired: 1 out]
          n242 = VISA Read(VISA resource name=w709, byte count=u32 15, error in (no error)=w711) -> (VISA resource name out=w714:refnum<visa-resource-name>, read buffer=w704:string, error out=w713:errorcluster)  [unwired: 1 out]
          n243 = String Subset(string=w704, length (rest)=8 ("offset (0)")) -> (substring=w706:string)  [unwired: 1 in]
          n244 = Equal?(x=w706, y=":TEC OFF") -> (x = y?=w701:bool)
          n245 = Not(x=w701) -> (.not. x?=w700:bool)
          n246 = Bundle By Name(cluster=w703, "WV Online TEC"=w700) -> (w702:T2)
        }
        frame "WV Online LD" {
          n247 = VISA Write(VISA resource name=w736, write buffer=w737, error in (no error)=w735) -> (VISA resource name out=w729:refnum<visa-resource-name>, error out=w731:errorcluster)  [unwired: 1 out]
          n248 = VISA Write(VISA resource name=w729, write buffer=":laser?", error in (no error)=w731) -> (VISA resource name out=w728:refnum<visa-resource-name>, error out=w730:errorcluster)  [unwired: 1 out]
          n249 = VISA Read(VISA resource name=w728, byte count=u32 15, error in (no error)=w730) -> (VISA resource name out=w733:refnum<visa-resource-name>, read buffer=w723:string, error out=w732:errorcluster)  [unwired: 1 out]
          n250 = String Subset(string=w723, length (rest)=10 ("offset (0)")) -> (substring=w725:string)  [unwired: 1 in]
          n251 = Equal?(x=w725, y=":LASER OFF") -> (x = y?=w720:bool)
          n252 = Not(x=w720) -> (.not. x?=w719:bool)
          n253 = Bundle By Name(cluster=w722, "WV Online LD"=w719) -> (w721:T2)
        }
        frame "WV Offline TEC" {
          n254 = VISA Write(VISA resource name=w755, write buffer=w756, error in (no error)=w754) -> (VISA resource name out=w748:refnum<visa-resource-name>, error out=w750:errorcluster)  [unwired: 1 out]
          n255 = VISA Write(VISA resource name=w748, write buffer=":tec?", error in (no error)=w750) -> (VISA resource name out=w747:refnum<visa-resource-name>, error out=w749:errorcluster)  [unwired: 1 out]
          n256 = VISA Read(VISA resource name=w747, byte count=u32 15, error in (no error)=w749) -> (VISA resource name out=w752:refnum<visa-resource-name>, read buffer=w742:string, error out=w751:errorcluster)  [unwired: 1 out]
          n257 = String Subset(string=w742, length (rest)=8 ("offset (0)")) -> (substring=w744:string)  [unwired: 1 in]
          n258 = Equal?(x=w744, y=":TEC OFF") -> (x = y?=w739:bool)
          n259 = Not(x=w739) -> (.not. x?=w738:bool)
          n260 = Bundle By Name(cluster=w741, "WV Offline TEC"=w738) -> (w740:T2)
        }
        frame "WV Offline LD" {
          n261 = VISA Write(VISA resource name=w774, write buffer=w775, error in (no error)=w773) -> (VISA resource name out=w767:refnum<visa-resource-name>, error out=w769:errorcluster)  [unwired: 1 out]
          n262 = VISA Write(VISA resource name=w767, write buffer=":laser?", error in (no error)=w769) -> (VISA resource name out=w766:refnum<visa-resource-name>, error out=w768:errorcluster)  [unwired: 1 out]
          n263 = VISA Read(VISA resource name=w766, byte count=u32 15, error in (no error)=w768) -> (VISA resource name out=w771:refnum<visa-resource-name>, read buffer=w761:string, error out=w770:errorcluster)  [unwired: 1 out]
          n264 = String Subset(string=w761, length (rest)=10 ("offset (0)")) -> (substring=w763:string)  [unwired: 1 in]
          n265 = Equal?(x=w763, y=":LASER OFF") -> (x = y?=w758:bool)
          n266 = Not(x=w758) -> (.not. x?=w757:bool)
          n267 = Bundle By Name(cluster=w760, "WV Offline LD"=w757) -> (w759:T2)
        }
        frame "WV Etalon TEC" {
          n268 = VISA Write(VISA resource name=w793, write buffer=w794, error in (no error)=w792) -> (VISA resource name out=w786:refnum<visa-resource-name>, error out=w788:errorcluster)  [unwired: 1 out]
          n269 = VISA Write(VISA resource name=w786, write buffer=":tec?", error in (no error)=w788) -> (VISA resource name out=w785:refnum<visa-resource-name>, error out=w787:errorcluster)  [unwired: 1 out]
          n270 = VISA Read(VISA resource name=w785, byte count=u32 15, error in (no error)=w787) -> (VISA resource name out=w790:refnum<visa-resource-name>, read buffer=w780:string, error out=w789:errorcluster)  [unwired: 1 out]
          n271 = String Subset(string=w780, length (rest)=8 ("offset (0)")) -> (substring=w782:string)  [unwired: 1 in]
          n272 = Equal?(x=w782, y=":TEC OFF") -> (x = y?=w777:bool)
          n273 = Not(x=w777) -> (.not. x?=w776:bool)
          n274 = Bundle By Name(cluster=w779, "WV Etalon TEC"=w776) -> (w778:T2)
        }
        frame "HSRL Etalon TEC" {
          n275 = VISA Write(VISA resource name=w812, write buffer=w813, error in (no error)=w811) -> (VISA resource name out=w805:refnum<visa-resource-name>, error out=w807:errorcluster)  [unwired: 1 out]
          n276 = VISA Write(VISA resource name=w805, write buffer=":tec?", error in (no error)=w807) -> (VISA resource name out=w804:refnum<visa-resource-name>, error out=w806:errorcluster)  [unwired: 1 out]
          n277 = VISA Read(VISA resource name=w804, byte count=u32 15, error in (no error)=w806) -> (VISA resource name out=w809:refnum<visa-resource-name>, read buffer=w799:string, error out=w808:errorcluster)  [unwired: 1 out]
          n278 = String Subset(string=w799, length (rest)=8 ("offset (0)")) -> (substring=w801:string)  [unwired: 1 in]
          n279 = Equal?(x=w801, y=":TEC OFF") -> (x = y?=w796:bool)
          n280 = Not(x=w796) -> (.not. x?=w795:bool)
          n281 = Bundle By Name(cluster=w798, "HSRL Etalon TEC"=w795) -> (w797:T2)
        }
        frame "HSRL TEC" {
          n282 = VISA Write(VISA resource name=w831, write buffer=w832, error in (no error)=w830) -> (VISA resource name out=w824:refnum<visa-resource-name>, error out=w826:errorcluster)  [unwired: 1 out]
          n283 = VISA Write(VISA resource name=w824, write buffer=":tec?", error in (no error)=w826) -> (VISA resource name out=w823:refnum<visa-resource-name>, error out=w825:errorcluster)  [unwired: 1 out]
          n284 = VISA Read(VISA resource name=w823, byte count=u32 15, error in (no error)=w825) -> (VISA resource name out=w828:refnum<visa-resource-name>, read buffer=w818:string, error out=w827:errorcluster)  [unwired: 1 out]
          n285 = String Subset(string=w818, length (rest)=8 ("offset (0)")) -> (substring=w820:string)  [unwired: 1 in]
          n286 = Equal?(x=w820, y=":TEC OFF") -> (x = y?=w815:bool)
          n287 = Not(x=w815) -> (.not. x?=w814:bool)
          n288 = Bundle By Name(cluster=w817, "HSRL TEC"=w814) -> (w816:T2)
        }
        frame "HSRL LD" {
          n289 = VISA Write(VISA resource name=w850, write buffer=w851, error in (no error)=w849) -> (VISA resource name out=w843:refnum<visa-resource-name>, error out=w845:errorcluster)  [unwired: 1 out]
          n290 = VISA Write(VISA resource name=w843, write buffer=":laser?", error in (no error)=w845) -> (VISA resource name out=w842:refnum<visa-resource-name>, error out=w844:errorcluster)  [unwired: 1 out]
          n291 = VISA Read(VISA resource name=w842, byte count=u32 15, error in (no error)=w844) -> (VISA resource name out=w847:refnum<visa-resource-name>, read buffer=w839:string, error out=w846:errorcluster)  [unwired: 1 out]
          n292 = String Subset(string=w839, length (rest)=10 ("offset (0)")) -> (substring=w841:string)  [unwired: 1 in]
          n293 = Equal?(x=w841, y=":LASER OFF") -> (x = y?=w836:bool)
          n294 = Not(x=w836) -> (.not. x?=w835:bool)
          n295 = Bundle By Name(cluster=w838, "HSRL LD"=w835) -> (w837:T2)
        }
      }
    }
    frame "Set_Limits" {
    }
    frame "Read_Limits" {
    }
    frame "Enable_Status" {
    }
    frame "Read_Status" {
      # "Read the on/off status, TEC set and actual temperatures and laser diode set and actual current and updates the front panel"
      n296 = for {
        tunnel: w871 -> [w879] mode=indexing
        tunnel: w870 -> [w880]
        tunnel: [w875] -> w866
        tunnel: w867 -> [w876]
        tunnel: [w877] -> w868
        shift-right: [w874] -> w864
        shift-left: w865 -> [w881]
        shift-right: [w873] -> _
        shift-left: w869 -> [w878]
        i -> [w882]
        n297 = case shown="2" w882 {
          tunnel: w881 -> [w895 w937 w973 w1015 w1051 w1090 w1129 w1169]
          tunnel: w876 -> [w898 w940 w976 w1018 w1054 w1093 w1132 w1172]
          tunnel: w880 -> [w897 w939 w975 w1017 w1053 w1092 w1131 w1171]
          tunnel: w879 -> [w896 w938 w974 w1016 w1052 w1091 w1130 w1170]
          tunnel: w878 -> [w892 w933 w969 w1011 w1047 w1086 w1125 w1165]
          tunnel: [w887 w928 w964 w1006 w1042 w1081 w1120 w1160] -> w877
          tunnel: [w886 w927 w963 w1005 w1041 w1080 w1119 w1159] -> w875
          tunnel: [w884 w922 w962 w1001 w1039 w1078 w1117 w1157] -> w874
          tunnel: [w885 w923 w961 w1000 w1040 w1079 w1118 w1158] -> w873
          frame 0, Default {
            n298 = Concatenate Strings(w896, ";:tec?" ("write buffer")) -> (w918:string)
            n299 = Concatenate Strings(w896, ";:temp:set?" ("write buffer")) -> (w905:string)
            n300 = Concatenate Strings(w896, ";:temp:act?" ("write buffer")) -> (w900:string)
            n301 = VISA Write(VISA resource name=w898, write buffer=w918, error in (no error)=w897) -> (VISA resource name out=w919:refnum<visa-resource-name>, error out=w920:errorcluster)  [unwired: 1 out]
            n302 = VISA Read(VISA resource name=w919, byte count=u32 30, error in (no error)=w920) -> (VISA resource name out=w909:refnum<visa-resource-name>, read buffer=w913:string, error out=w908:errorcluster)  [unwired: 1 out]
            n303 = String Subset(string=w913, length (rest)=7 ("offset (0)")) -> (substring=w915:string)  [unwired: 1 in]
            n304 = VISA Write(VISA resource name=w909, write buffer=w905, error in (no error)=w908) -> (VISA resource name out=w910:refnum<visa-resource-name>, error out=w911:errorcluster)  [unwired: 1 out]
            n305 = Equal?(x=w915, y=":TEC ON") -> (x = y?=w883:bool)
            n306 = VISA Read(VISA resource name=w910, byte count=u32 30, error in (no error)=w911) -> (VISA resource name out=w901:refnum<visa-resource-name>, read buffer=w893:string, error out=w902:errorcluster)  [unwired: 1 out]
            n307 = Fract/Exp String To Number(string=w893, offset=10) -> (number=w888:dbl)  [unwired: 2 in, 1 out]
            n308 = VISA Write(VISA resource name=w901, write buffer=w900, error in (no error)=w902) -> (VISA resource name out=w903:refnum<visa-resource-name>, error out=w899:errorcluster)  [unwired: 1 out]
            n309 = VISA Read(VISA resource name=w903, byte count=u32 30, error in (no error)=w899) -> (VISA resource name out=w887:refnum<visa-resource-name>, read buffer=w890:string, error out=w886:errorcluster)  [unwired: 1 out]
            n310 = Fract/Exp String To Number(string=w890, offset=10) -> (number=w889:dbl)  [unwired: 2 in, 1 out]
            n311 = Bundle By Name(cluster=w892, "WV Online TEC"=w888) -> (w885:T3)
            n312 = Bundle By Name(cluster=w895, "WV OnLine TEC"=w889, "WV Online TEC"=w883, "Pro8000"=w883) -> (w884:T2)
            n313 = local write "Readings"(w884) -> ()
            n314 = local write "Settings"(w885) -> ()
          }
          frame 1 {
            n315 = Concatenate Strings(w938, ";:laser?" ("write buffer")) -> (w957:string)
            n316 = Concatenate Strings(w938, ";:ild:set?" ("write buffer")) -> (w947:string)
            n317 = Concatenate Strings(w938, ";:ild:act?" ("write buffer")) -> (w942:string)
            n318 = VISA Write(VISA resource name=w940, write buffer=w957, error in (no error)=w939) -> (VISA resource name out=w958:refnum<visa-resource-name>, error out=w959:errorcluster)  [unwired: 1 out]
            n319 = VISA Read(VISA resource name=w958, byte count=u32 30, error in (no error)=w959) -> (VISA resource name out=w949:refnum<visa-resource-name>, read buffer=w953:string, error out=w948:errorcluster)  [unwired: 1 out]
            n320 = String Subset(string=w953, length (rest)=9 ("offset (0)")) -> (substring=w955:string)  [unwired: 1 in]
            n321 = VISA Write(VISA resource name=w949, write buffer=w947, error in (no error)=w948) -> (VISA resource name out=w950:refnum<visa-resource-name>, error out=w951:errorcluster)  [unwired: 1 out]
            n322 = Equal?(x=w955, y=":LASER ON") -> (x = y?=w936:bool)
            n323 = VISA Read(VISA resource name=w950, byte count=u32 30, error in (no error)=w951) -> (VISA resource name out=w943:refnum<visa-resource-name>, read buffer=w934:string, error out=w944:errorcluster)  [unwired: 1 out]
            n324 = Fract/Exp String To Number(string=w934, offset=9) -> (number=w929:dbl)  [unwired: 2 in, 1 out]
            n325 = VISA Write(VISA resource name=w943, write buffer=w942, error in (no error)=w944) -> (VISA resource name out=w945:refnum<visa-resource-name>, error out=w941:errorcluster)  [unwired: 1 out]
            n326 = VISA Read(VISA resource name=w945, byte count=u32 30, error in (no error)=w941) -> (VISA resource name out=w928:refnum<visa-resource-name>, read buffer=w931:string, error out=w927:errorcluster)  [unwired: 1 out]
            n327 = Fract/Exp String To Number(string=w931, offset=9) -> (number=w930:dbl)  [unwired: 2 in, 1 out]
            n328 = Bundle By Name(cluster=w933, "WV Online LD"=w929) -> (w923:T3)
            n329 = Bundle By Name(cluster=w937, "WV Online LD"=w930, "WV Online LD"=w936) -> (w922:T2)
            n330 = local write "Readings"(w922) -> ()
            n331 = local write "Settings"(w923) -> ()
          }
          frame 2 {
            n332 = Concatenate Strings(w974, ";:tec?" ("write buffer")) -> (w996:string)
            n333 = Concatenate Strings(w974, ";:temp:set?" ("write buffer")) -> (w983:string)
            n334 = Concatenate Strings(w974, ";:temp:act?" ("write buffer")) -> (w978:string)
            n335 = VISA Write(VISA resource name=w976, write buffer=w996, error in (no error)=w975) -> (VISA resource name out=w997:refnum<visa-resource-name>, error out=w998:errorcluster)  [unwired: 1 out]
            n336 = VISA Read(VISA resource name=w997, byte count=u32 30, error in (no error)=w998) -> (VISA resource name out=w987:refnum<visa-resource-name>, read buffer=w991:string, error out=w986:errorcluster)  [unwired: 1 out]
            n337 = String Subset(string=w991, length (rest)=7 ("offset (0)")) -> (substring=w993:string)  [unwired: 1 in]
            n338 = VISA Write(VISA resource name=w987, write buffer=w983, error in (no error)=w986) -> (VISA resource name out=w988:refnum<visa-resource-name>, error out=w989:errorcluster)  [unwired: 1 out]
            n339 = Equal?(x=w993, y=":TEC ON") -> (x = y?=w972:bool)
            n340 = VISA Read(VISA resource name=w988, byte count=u32 30, error in (no error)=w989) -> (VISA resource name out=w979:refnum<visa-resource-name>, read buffer=w970:string, error out=w980:errorcluster)  [unwired: 1 out]
            n341 = Fract/Exp String To Number(string=w970, offset=10) -> (number=w965:dbl)  [unwired: 2 in, 1 out]
            n342 = VISA Write(VISA resource name=w979, write buffer=w978, error in (no error)=w980) -> (VISA resource name out=w981:refnum<visa-resource-name>, error out=w977:errorcluster)  [unwired: 1 out]
            n343 = VISA Read(VISA resource name=w981, byte count=u32 30, error in (no error)=w977) -> (VISA resource name out=w964:refnum<visa-resource-name>, read buffer=w967:string, error out=w963:errorcluster)  [unwired: 1 out]
            n344 = Fract/Exp String To Number(string=w967, offset=10) -> (number=w966:dbl)  [unwired: 2 in, 1 out]
            n345 = Bundle By Name(cluster=w969, "WV Offline TEC"=w965) -> (w961:T3)
            n346 = Bundle By Name(cluster=w973, "WV Offline TEC"=w966, "WV Offline TEC"=w972) -> (w962:T2)
            n347 = local write "Readings"(w962) -> ()
            n348 = local write "Settings"(w961) -> ()
          }
          frame 3 {
            n349 = Concatenate Strings(w1016, ";:laser?" ("write buffer")) -> (w1035:string)
            n350 = Concatenate Strings(w1016, ";:ild:set?" ("write buffer")) -> (w1025:string)
            n351 = Concatenate Strings(w1016, ";:ild:act?" ("write buffer")) -> (w1020:string)
            n352 = VISA Write(VISA resource name=w1018, write buffer=w1035, error in (no error)=w1017) -> (VISA resource name out=w1036:refnum<visa-resource-name>, error out=w1037:errorcluster)  [unwired: 1 out]
            n353 = VISA Read(VISA resource name=w1036, byte count=u32 30, error in (no error)=w1037) -> (VISA resource name out=w1027:refnum<visa-resource-name>, read buffer=w1031:string, error out=w1026:errorcluster)  [unwired: 1 out]
            n354 = String Subset(string=w1031, length (rest)=9 ("offset (0)")) -> (substring=w1033:string)  [unwired: 1 in]
            n355 = VISA Write(VISA resource name=w1027, write buffer=w1025, error in (no error)=w1026) -> (VISA resource name out=w1028:refnum<visa-resource-name>, error out=w1029:errorcluster)  [unwired: 1 out]
            n356 = Equal?(x=w1033, y=":LASER ON") -> (x = y?=w1014:bool)
            n357 = VISA Read(VISA resource name=w1028, byte count=u32 30, error in (no error)=w1029) -> (VISA resource name out=w1021:refnum<visa-resource-name>, read buffer=w1012:string, error out=w1022:errorcluster)  [unwired: 1 out]
            n358 = Fract/Exp String To Number(string=w1012, offset=9) -> (number=w1007:dbl)  [unwired: 2 in, 1 out]
            n359 = VISA Write(VISA resource name=w1021, write buffer=w1020, error in (no error)=w1022) -> (VISA resource name out=w1023:refnum<visa-resource-name>, error out=w1019:errorcluster)  [unwired: 1 out]
            n360 = VISA Read(VISA resource name=w1023, byte count=u32 30, error in (no error)=w1019) -> (VISA resource name out=w1006:refnum<visa-resource-name>, read buffer=w1009:string, error out=w1005:errorcluster)  [unwired: 1 out]
            n361 = Fract/Exp String To Number(string=w1009, offset=9) -> (number=w1008:dbl)  [unwired: 2 in, 1 out]
            n362 = Bundle By Name(cluster=w1011, "WV Offline LD"=w1007) -> (w1000:T3)
            n363 = Bundle By Name(cluster=w1015, "WV Offline LD"=w1008, "WV Offline LD"=w1014) -> (w1001:T2)
            n364 = local write "Readings"(w1001) -> ()
            n365 = local write "Settings"(w1000) -> ()
          }
          frame 4 {
            n366 = Concatenate Strings(w1052, ";:tec?" ("write buffer")) -> (w1074:string)
            n367 = Concatenate Strings(w1052, ";:temp:set?" ("write buffer")) -> (w1061:string)
            n368 = Concatenate Strings(w1052, ";:temp:act?" ("write buffer")) -> (w1056:string)
            n369 = VISA Write(VISA resource name=w1054, write buffer=w1074, error in (no error)=w1053) -> (VISA resource name out=w1075:refnum<visa-resource-name>, error out=w1076:errorcluster)  [unwired: 1 out]
            n370 = VISA Read(VISA resource name=w1075, byte count=u32 30, error in (no error)=w1076) -> (VISA resource name out=w1065:refnum<visa-resource-name>, read buffer=w1069:string, error out=w1064:errorcluster)  [unwired: 1 out]
            n371 = String Subset(string=w1069, length (rest)=7 ("offset (0)")) -> (substring=w1071:string)  [unwired: 1 in]
            n372 = VISA Write(VISA resource name=w1065, write buffer=w1061, error in (no error)=w1064) -> (VISA resource name out=w1066:refnum<visa-resource-name>, error out=w1067:errorcluster)  [unwired: 1 out]
            n373 = Equal?(x=w1071, y=":TEC ON") -> (x = y?=w1050:bool)
            n374 = VISA Read(VISA resource name=w1066, byte count=u32 30, error in (no error)=w1067) -> (VISA resource name out=w1057:refnum<visa-resource-name>, read buffer=w1048:string, error out=w1058:errorcluster)  [unwired: 1 out]
            n375 = Fract/Exp String To Number(string=w1048, offset=10) -> (number=w1043:dbl)  [unwired: 2 in, 1 out]
            n376 = VISA Write(VISA resource name=w1057, write buffer=w1056, error in (no error)=w1058) -> (VISA resource name out=w1059:refnum<visa-resource-name>, error out=w1055:errorcluster)  [unwired: 1 out]
            n377 = VISA Read(VISA resource name=w1059, byte count=u32 30, error in (no error)=w1055) -> (VISA resource name out=w1042:refnum<visa-resource-name>, read buffer=w1045:string, error out=w1041:errorcluster)  [unwired: 1 out]
            n378 = Fract/Exp String To Number(string=w1045, offset=10) -> (number=w1044:dbl)  [unwired: 2 in, 1 out]
            n379 = Bundle By Name(cluster=w1047, "WV Etalon TEC"=w1043) -> (w1040:T3)
            n380 = Bundle By Name(cluster=w1051, "WV EtalonTEC"=w1044, "WV Etalon TEC"=w1050) -> (w1039:T2)
            n381 = local write "Readings"(w1039) -> ()
            n382 = local write "Settings"(w1040) -> ()
          }
          frame 5 {
            n383 = Concatenate Strings(w1091, ";:tec?" ("write buffer")) -> (w1113:string)
            n384 = Concatenate Strings(w1091, ";:temp:set?" ("write buffer")) -> (w1100:string)
            n385 = Concatenate Strings(w1091, ";:temp:act?" ("write buffer")) -> (w1095:string)
            n386 = VISA Write(VISA resource name=w1093, write buffer=w1113, error in (no error)=w1092) -> (VISA resource name out=w1114:refnum<visa-resource-name>, error out=w1115:errorcluster)  [unwired: 1 out]
            n387 = VISA Read(VISA resource name=w1114, byte count=u32 30, error in (no error)=w1115) -> (VISA resource name out=w1104:refnum<visa-resource-name>, read buffer=w1108:string, error out=w1103:errorcluster)  [unwired: 1 out]
            n388 = String Subset(string=w1108, length (rest)=7 ("offset (0)")) -> (substring=w1110:string)  [unwired: 1 in]
            n389 = VISA Write(VISA resource name=w1104, write buffer=w1100, error in (no error)=w1103) -> (VISA resource name out=w1105:refnum<visa-resource-name>, error out=w1106:errorcluster)  [unwired: 1 out]
            n390 = Equal?(x=w1110, y=":TEC ON") -> (x = y?=w1089:bool)
            n391 = VISA Read(VISA resource name=w1105, byte count=u32 30, error in (no error)=w1106) -> (VISA resource name out=w1096:refnum<visa-resource-name>, read buffer=w1087:string, error out=w1097:errorcluster)  [unwired: 1 out]
            n392 = Fract/Exp String To Number(string=w1087, offset=10) -> (number=w1082:dbl)  [unwired: 2 in, 1 out]
            n393 = VISA Write(VISA resource name=w1096, write buffer=w1095, error in (no error)=w1097) -> (VISA resource name out=w1098:refnum<visa-resource-name>, error out=w1094:errorcluster)  [unwired: 1 out]
            n394 = VISA Read(VISA resource name=w1098, byte count=u32 30, error in (no error)=w1094) -> (VISA resource name out=w1081:refnum<visa-resource-name>, read buffer=w1084:string, error out=w1080:errorcluster)  [unwired: 1 out]
            n395 = Fract/Exp String To Number(string=w1084, offset=10) -> (number=w1083:dbl)  [unwired: 2 in, 1 out]
            n396 = Bundle By Name(cluster=w1086, "HSRL Etalon TEC"=w1082) -> (w1079:T3)
            n397 = Bundle By Name(cluster=w1090, "HSRL Etalon TEC"=w1083, "HSRL Etalon TEC"=w1089) -> (w1078:T2)
            n398 = local write "Readings"(w1078) -> ()
            n399 = local write "Settings"(w1079) -> ()
          }
          frame 6 {
            n400 = Concatenate Strings(w1130, ";:tec?" ("write buffer")) -> (w1152:string)
            n401 = Concatenate Strings(w1130, ";:temp:set?" ("write buffer")) -> (w1139:string)
            n402 = Concatenate Strings(w1130, ";:temp:act?" ("write buffer")) -> (w1134:string)
            n403 = VISA Write(VISA resource name=w1132, write buffer=w1152, error in (no error)=w1131) -> (VISA resource name out=w1153:refnum<visa-resource-name>, error out=w1154:errorcluster)  [unwired: 1 out]
            n404 = VISA Read(VISA resource name=w1153, byte count=u32 30, error in (no error)=w1154) -> (VISA resource name out=w1143:refnum<visa-resource-name>, read buffer=w1147:string, error out=w1142:errorcluster)  [unwired: 1 out]
            n405 = String Subset(string=w1147, length (rest)=7 ("offset (0)")) -> (substring=w1149:string)  [unwired: 1 in]
            n406 = VISA Write(VISA resource name=w1143, write buffer=w1139, error in (no error)=w1142) -> (VISA resource name out=w1144:refnum<visa-resource-name>, error out=w1145:errorcluster)  [unwired: 1 out]
            n407 = Equal?(x=w1149, y=":TEC ON") -> (x = y?=w1128:bool)
            n408 = VISA Read(VISA resource name=w1144, byte count=u32 30, error in (no error)=w1145) -> (VISA resource name out=w1135:refnum<visa-resource-name>, read buffer=w1126:string, error out=w1136:errorcluster)  [unwired: 1 out]
            n409 = Fract/Exp String To Number(string=w1126, offset=10) -> (number=w1121:dbl)  [unwired: 2 in, 1 out]
            n410 = VISA Write(VISA resource name=w1135, write buffer=w1134, error in (no error)=w1136) -> (VISA resource name out=w1137:refnum<visa-resource-name>, error out=w1133:errorcluster)  [unwired: 1 out]
            n411 = VISA Read(VISA resource name=w1137, byte count=u32 30, error in (no error)=w1133) -> (VISA resource name out=w1120:refnum<visa-resource-name>, read buffer=w1123:string, error out=w1119:errorcluster)  [unwired: 1 out]
            n412 = Fract/Exp String To Number(string=w1123, offset=10) -> (number=w1122:dbl)  [unwired: 2 in, 1 out]
            n413 = Bundle By Name(cluster=w1129, "HSRL TEC"=w1122, "HSRL TEC"=w1128) -> (w1117:T2)
            n414 = Bundle By Name(cluster=w1125, "HSRL TEC"=w1121) -> (w1118:T3)
            n415 = local write "Readings"(w1117) -> ()
            n416 = local write "Settings"(w1118) -> ()
          }
          frame 7 {
            n417 = Concatenate Strings(w1170, ";:laser?" ("write buffer")) -> (w1191:string)
            n418 = Concatenate Strings(w1170, ";:ild:set?" ("write buffer")) -> (w1179:string)
            n419 = Concatenate Strings(w1170, ";:ild:act?" ("write buffer")) -> (w1174:string)
            n420 = VISA Write(VISA resource name=w1172, write buffer=w1191, error in (no error)=w1171) -> (VISA resource name out=w1192:refnum<visa-resource-name>, error out=w1193:errorcluster)  [unwired: 1 out]
            n421 = VISA Read(VISA resource name=w1192, byte count=u32 30, error in (no error)=w1193) -> (VISA resource name out=w1183:refnum<visa-resource-name>, read buffer=w1187:string, error out=w1182:errorcluster)  [unwired: 1 out]
            n422 = String Subset(string=w1187, length (rest)=9 ("offset (0)")) -> (substring=w1189:string)  [unwired: 1 in]
            n423 = VISA Write(VISA resource name=w1183, write buffer=w1179, error in (no error)=w1182) -> (VISA resource name out=w1184:refnum<visa-resource-name>, error out=w1185:errorcluster)  [unwired: 1 out]
            n424 = Equal?(x=w1189, y=":LASER ON") -> (x = y?=w1168:bool)
            n425 = VISA Read(VISA resource name=w1184, byte count=u32 30, error in (no error)=w1185) -> (VISA resource name out=w1175:refnum<visa-resource-name>, read buffer=w1166:string, error out=w1176:errorcluster)  [unwired: 1 out]
            n426 = Fract/Exp String To Number(string=w1166, offset=9) -> (number=w1161:dbl)  [unwired: 2 in, 1 out]
            n427 = VISA Write(VISA resource name=w1175, write buffer=w1174, error in (no error)=w1176) -> (VISA resource name out=w1177:refnum<visa-resource-name>, error out=w1173:errorcluster)  [unwired: 1 out]
            n428 = VISA Read(VISA resource name=w1177, byte count=u32 30, error in (no error)=w1173) -> (VISA resource name out=w1160:refnum<visa-resource-name>, read buffer=w1163:string, error out=w1159:errorcluster)  [unwired: 1 out]
            n429 = Fract/Exp String To Number(string=w1163, offset=9) -> (number=w1162:dbl)  [unwired: 2 in, 1 out]
            n430 = Bundle By Name(cluster=w1165, "HSRL LD"=w1161) -> (w1158:T3)
            n431 = Bundle By Name(cluster=w1169, "HSRL LD"=w1162, "HSRL LD"=w1168) -> (w1157:T2)
            n432 = local write "Readings"(w1157) -> ()
            n433 = local write "Settings"(w1158) -> ()
          }
        }
      }
    }
  }
  "error out" <- w17
  "Device Out" <- w13
  "Response" <- w12
  "Readings" <- w3
